vi "get_config_cluster.vi"(8 "error in (no error)":errorcluster, 11 "LightSourceAN191011Chameleon in":refnum<class "LightSourceAN191011Chameleon.lvclass">) -> (0 "error out":errorcluster, 2 "config cluster (variant)":variant, 3 "LightSourceAN191011Chameleon out":refnum<class "LightSourceAN191011Chameleon.lvclass">)   [LabVIEW 2010, in "LightSourceAN191011Chameleon.lvclass"]
uses:
  LightSourceAN191011Chameleon.lvclass
  LightSourceAN191011Chameleon.lvclass/LightSourceAN191011Chameleon.ctl
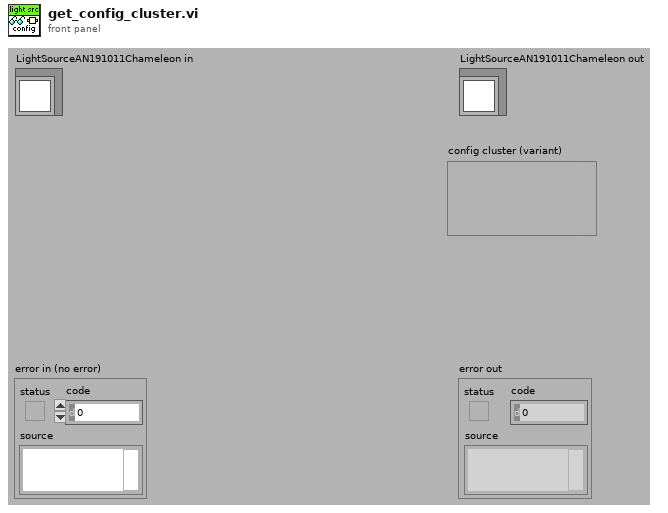
[diagram p1: front panel]
types:
  T1 = typedef "LightSourceAN191011Chameleon.lvclass/config_data.ctl" = cluster{"communication settings":cluster{"comm port":string, "data bits":u16, "parity":enum16{"None", "Odd", "Even", "Mark", "Space"}, "baud rate":u32, "delay before read":u32, "stop bits":u16}, "laser settings":cluster{"start wavelength":dbl[unit]}}
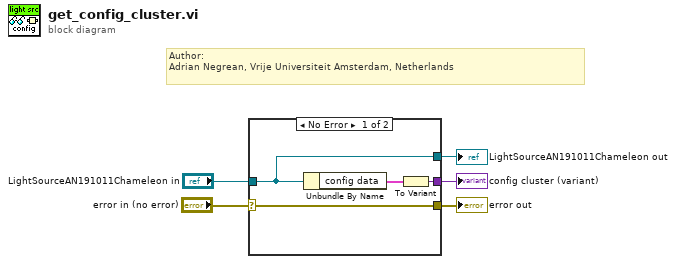
[diagram p0: block diagram]
diagram:
  # "Author: \nAdrian Negrean, Vrije Universiteit Amsterdam, Netherlands"
  n1 = case shown="No Error" "error in (no error)" {
    selector: "error in (no error)" -> [w9 w11]
    tunnel: [w9 w11] -> w4
    tunnel: "LightSourceAN191011Chameleon in" -> [w6 w10]
    tunnel: [w7 _] -> w2
    tunnel: [w6 w10] -> w1
    frame No Error {
      n2 = Unbundle By Name(w6) -> ("config data"=w8:T1)
      n3 = To Variant(anything=w8) -> (Variant=w7:variant)
    }
    frame Error {
    }
  }
  "error out" <- w4
  "LightSourceAN191011Chameleon out" <- w1
  "config cluster (variant)" <- w2
